vi "GRNF_GenericSolenoid.vi"(7 "RefNum Name":string="My Motor RefNum") -> (0 "Error":errorcluster, 3 "Device Reference":T1={"DevStatus"={"status"=FALSE, "code"=0, "source"=""}, "Pneumatics Control Module"=0, "Forward Solenoid Channel"=enum."Invalid", "Reverse Solenoid Channel"=enum."Invalid"})   [LabVIEW 2019]
uses:
  <vilib>/Rock Robotics/WPI/Solenoid/WPI_SolenoidDevRef.ctl
  <vilib>/Rock Robotics/WPI/Solenoid/WPI_SolenoidChannel.ctl
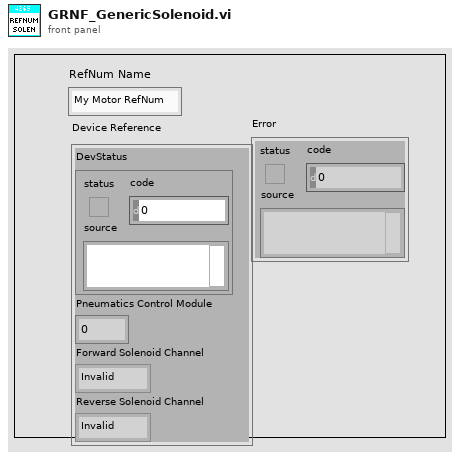
[diagram p1: front panel]
types:
  T1 = typedef "WPI_SolenoidDevRef.ctl" = cluster{"DevStatus":errorcluster, "Pneumatics Control Module":u8, "Forward Solenoid Channel":T2, "Reverse Solenoid Channel":T2}
  T2 = typedef "WPI_SolenoidChannel.ctl" = enum8{"Solenoid 0", "Solenoid 1", "Solenoid 2", "Solenoid 3", "Solenoid 4", "Solenoid 5", "Solenoid 6", "Solenoid 7", "Invalid"}
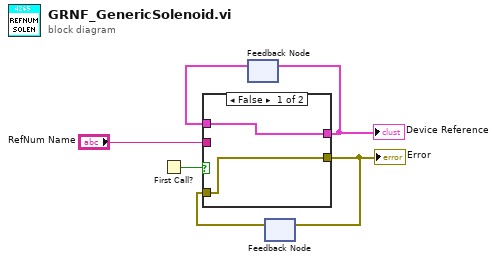
[diagram p0: block diagram]
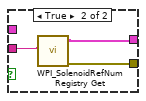
[diagram p2: hidden frame]
diagram:
  n1 = First Call?() -> (First Call?: T/F=w6:bool)
  n2 = feedback #1() -> (w5:T1)  [unwired: 1 in]
  n3 = feedback #2() -> (w1:errorcluster)  [unwired: 1 in]
  n4 = case shown="False" w6 {
    tunnel: [w8 w10] -> w4
    tunnel: w5 -> [w8 _]
    tunnel: "RefNum Name" -> [_ w11]
    tunnel: [w7 w9] -> w2
    tunnel: w1 -> [w7 _]
    frame False {
    }
    frame True {
      n5 = call <vilib>:"WPI_SolenoidRefNum Registry Get.vi"("refnum name"=w11) -> ("error out"=w9:errorcluster, "SolenoidDevRef"=w10:T1)  [unwired: 9 in]
    }
  }
  "Device Reference" <- w4
  "Error" <- w2
  n6 = feedback-in #1(w4) -> ()
  n7 = feedback-in #2(w2) -> ()
